vi "Tree-DeleteItems.vi"(8 "error In":errorcluster, 10 "All Tags":string[](array[string]), 11 "Tree In":refnum<vi>) -> (0 "error out":errorcluster, 3 "Tree out":refnum<vi>)   [LabVIEW 2013]
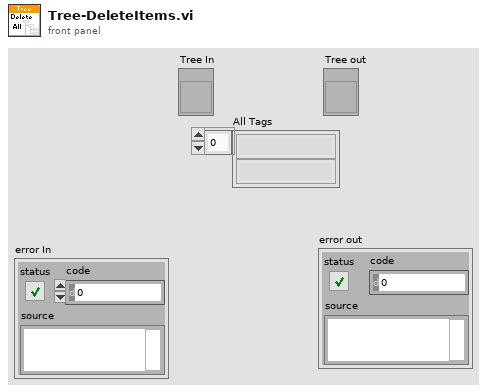
[diagram p1: front panel]
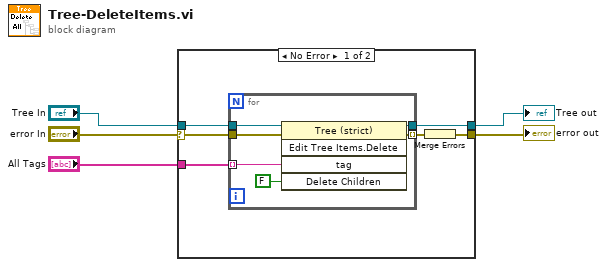
[diagram p0: block diagram]
diagram:
  n1 = case shown="No Error" "error In" {
    selector: "error In" -> [w8 w18]
    tunnel: [w11 w19] -> w5
    tunnel: "Tree In" -> [w10 w19]
    tunnel: "All Tags" -> [w9 _]
    tunnel: [w6 w18] -> w1
    frame No Error {
      n2 = for {
        tunnel: w9 -> [w16] mode=indexing
        tunnel: w10 -> [w15]
        tunnel: [w14] -> w11
        tunnel: w8 -> [w13]
        tunnel: [w12] -> w7 mode=indexing
        n3 = invoke class="Tree (strict)" method="Edit Tree Items.Delete"(reference=w15, error in=w13, "tag"=w16, "Delete Children"=FALSE ("Delete Children?")) -> (reference out=w14:refnum<vi>, error out=w12:errorcluster)  [unwired: 1 in, 3 out]
      }
      n4 = Merge Errors(w7) -> (w6:errorcluster)
    }
    frame Error {
    }
  }
  "Tree out" <- w5
  "error out" <- w1
